vi "MassCompile.vi"   [LabVIEW 2016, in "Script.lvlib"]
uses:
  Script.lvlib
  <vilib>/Wiresmith Technology/G CLI/Argument Parser/Option Class/Option Configuration.ctl
  <vilib>/Wiresmith Technology/G CLI/Argument Parser/Option Class/Argument Type.ctl
  <vilib>/Wiresmith Technology/G CLI/CLI Class/CLI.lvclass
  <vilib>/Wiresmith Technology/G CLI/Argument Parser/Option Class/Option.lvclass
  <vilib>/Wiresmith Technology/G CLI/Argument Parser/Option Set Class/Option Set.lvclass
types:
  T1 = typedef "Option Parser.lvlib/Option.lvclass/Option Configuration.ctl" = cluster{"Option Type":T2, "Option Labels":string[], "Key":string, "Description":string, "Required":bool, "Default Value":string}
  T2 = typedef "Option Parser.lvlib/Option.lvclass/Argument Type.ctl" = enum16{"flag", "value"}
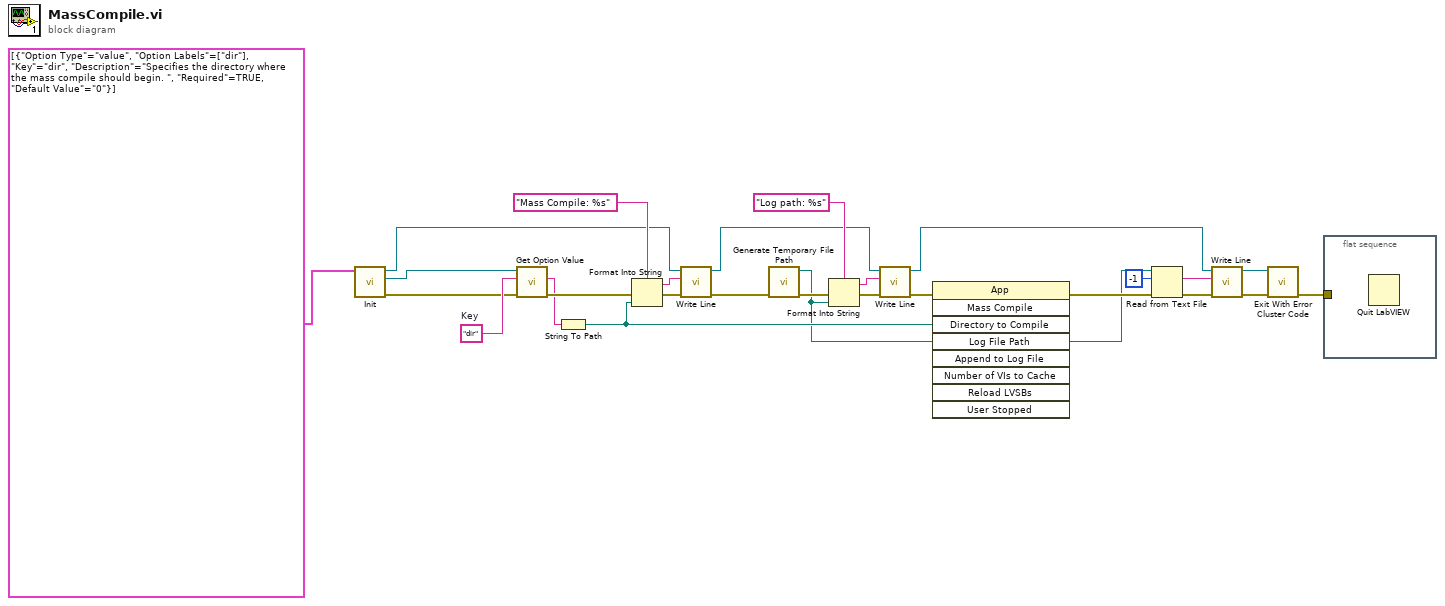
[diagram p0: block diagram]
diagram:
  w27 = "dir"  # Key
  n1 = call "Init.vi"("Options"=T1[] [{"Option Type"=enum."value", "Option Labels"=["dir"], "Key"="dir", "Description"="Specifies the directory where the mass compile should begin. ", "Required"=TRUE, "Default Value"="0"}]) -> ("error out"=w4:errorcluster, "Option Set out"=w2:refnum<class "Option Set.lvclass">, "CLI out"=w3:refnum<class "CLI.lvclass">)  [unwired: 8 in]
  n2 = call <vilib>:"Get Option Value.vi"("error in (no error)"=w4, "Option Key"=w27, "Option Set in"=w2) -> ("error out"=w20:errorcluster, "Value"=w16:string)  [unwired: 5 in, 2 out]
  n3 = String To Path(string=w16) -> (path=w15:path)
  n4 = Format Into String(format string="Mass Compile: %s", error in=w20, w15) -> (resulting string=w14:string, error out=w19:errorcluster)  [unwired: 1 in]
  n5 = call <vilib>:"Write Line.vi"("error in (no error)"=w19, "Text to Write"=w14, "CLI in"=w3) -> ("error out"=w25:errorcluster, "CLI out"=w17:refnum<class "CLI.lvclass">)  [unwired: 7 in]
  n6 = call <vilib>:"Generate Temporary File Path.vi"("error in (no error)"=w25) -> ("error out"=w23:errorcluster, "Unique Temporary File Path"=w11:path)  [unwired: 9 in]
  n7 = Format Into String(format string="Log path: %s", error in=w23, w11) -> (resulting string=w13:string, error out=w22:errorcluster)  [unwired: 1 in]
  n8 = call <vilib>:"Write Line.vi"("error in (no error)"=w22, "Text to Write"=w13, "CLI in"=w17) -> ("error out"=w24:errorcluster, "CLI out"=w8:refnum<class "CLI.lvclass">)  [unwired: 7 in]
  n9 = invoke class="App" method="Mass Compile"(error in=w24, "Directory to Compile"=w15, "Log File Path"=w11) -> (error out=w12:errorcluster)  [unwired: 6 in, 8 out]
  n10 = Read from Text File(file (use dialog)=w11, count=-1, error in=w12) -> (text=w9:string, error out=w7:errorcluster)  [unwired: 1 in, 2 out]
  n11 = call <vilib>:"Write Line.vi"("error in (no error)"=w7, "Text to Write"=w9, "CLI in"=w8) -> ("error out"=w6:errorcluster, "CLI out"=w5:refnum<class "CLI.lvclass">)  [unwired: 7 in]
  n12 = call <vilib>:"Exit With Error Cluster Code.vi"("error in (no error)"=w6, "CLI in"=w5) -> ("error out"=w26:errorcluster)  [unwired: 9 in]
  n13 = flat-sequence {
    tunnel: w26 -> [_]
    frame #0 {
      n14 = Quit LabVIEW() -> ()  [unwired: 1 in]
    }
  }
